vi "FIT Util Make Row 80 characters.vi"(11 "Row":string) -> (3 "Row with 80 char":string)   [LabVIEW 2024]
panel:
  out "length":i32
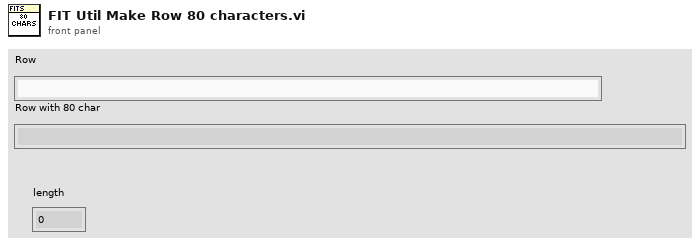
[diagram p1: front panel]
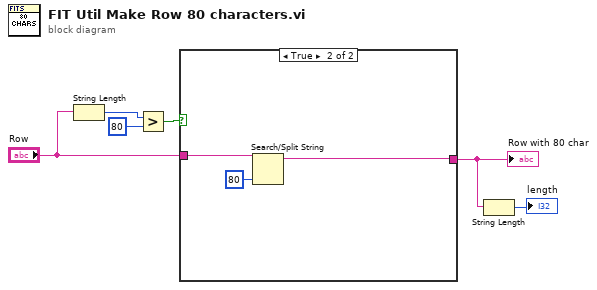
[diagram p0: block diagram]
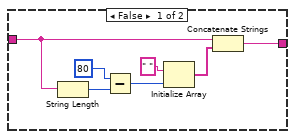
[diagram p2: hidden frame]
diagram:
  n1 = String Length(string="Row") -> (length=w3:i32)
  n2 = Greater?(x=w3, y=80) -> (0:w1:bool)
  n3 = case shown="True" w1 {
    tunnel: [w8 w14] -> w6
    tunnel: "Row" -> [w7 w16]
    frame False {
      n4 = String Length(string=w7) -> (length=w13:i32)
      n5 = Subtract(x=80, y=w13) -> (x-y=w10:i32)
      n6 = Initialize Array(" ", w10) -> (w9:string[])
      n7 = Concatenate Strings(w7, w9) -> (w8:string)
    }
    frame True {
      n8 = Search/Split String(string=w16, offset (0)=80) -> (substring before match=w14:string)  [unwired: 1 in, 2 out]
    }
  }
  "Row with 80 char" <- w6
  n9 = String Length(string=w6) -> (length=→"length":i32)
